vi "CalcLo.vi"(0 "dvotAFTKinetics in":refnum<class "dvotAFTKinetics.lvclass">, 1 "kParNum":i32, 2 "etchType":i32, 3 "kParValue":dbl, 4 "doProject":bool, 5 "error in (no error)":errorcluster) -> (14 "dvotAFTKinetics out":refnum<class "dvotAFTKinetics.lvclass">, 15 "Numeric":dbl, 19 "error out":errorcluster)   [LabVIEW 2012, in "dvotAFTKinetics.lvclass"]
uses:
  dvotAFTKinetics.lvclass
  dvotAFTKinetics.lvclass/dvotAFTKinetics.ctl
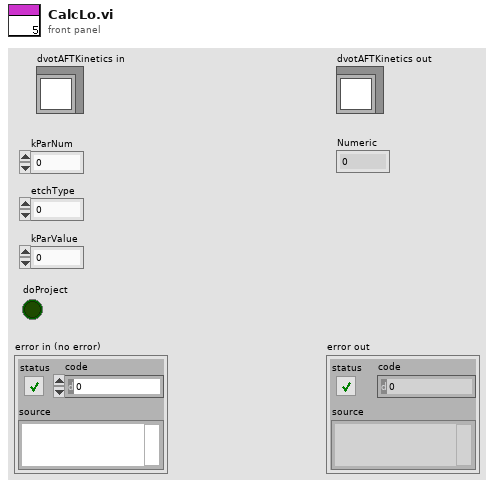
[diagram p1: front panel]
types:
  T1 = cluster{"lomSlope":dbl, "lomInt":dbl, "locSlope":dbl, "locInt":dbl}[]
  T2 = cluster{"lomSlope":dbl, "lomInt":dbl, "locSlope":dbl, "locInt":dbl}
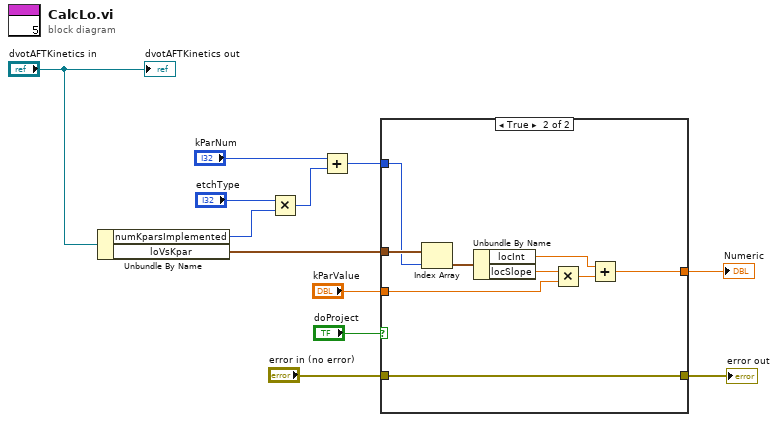
[diagram p0: block diagram]
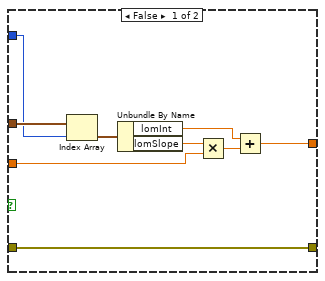
[diagram p2: hidden frame]
diagram:
  n1 = Unbundle By Name("dvotAFTKinetics in") -> ("numKparsImplemented"=w9:i32, "loVsKpar"=w5:T1)
  n2 = Multiply(x="etchType", y=w9) -> (x*y=w8:i32)
  n3 = Add(x="kParNum", y=w8) -> (x+y=w7:i32)
  n4 = case shown="True" "doProject" {
    tunnel: w7 -> [w16 w29]
    tunnel: "kParValue" -> [w15 w26]
    tunnel: w5 -> [w17 w30]
    tunnel: "error in (no error)" -> [w13 w22]
    tunnel: [w14 w23] -> w3
    tunnel: [w13 w22] -> w2
    frame False {
      n5 = Index Array(array=w17, index=w16) -> (element=w21:T2)
      n6 = Unbundle By Name(w21) -> ("lomInt"=w18:dbl, "lomSlope"=w20:dbl)
      n7 = Multiply(x=w20, y=w15) -> (x*y=w19:dbl)
      n8 = Add(x=w18, y=w19) -> (x+y=w14:dbl)
    }
    frame True {
      n9 = Index Array(array=w30, index=w29) -> (element=w28:T2)
      n10 = Unbundle By Name(w28) -> ("locInt"=w24:dbl, "locSlope"=w27:dbl)
      n11 = Multiply(x=w27, y=w26) -> (x*y=w25:dbl)
      n12 = Add(x=w24, y=w25) -> (x+y=w23:dbl)
    }
  }
  "error out" <- w2
  "Numeric" <- w3
  "dvotAFTKinetics out" <- "dvotAFTKinetics in"
